vi "CalculateScaleAndPositionToCenterImage.vi"(0 "reference in":refnum<class "LcPictureBox.lvclass">, 2 "ImageFile":path, 3 "Image":refnum<k24>, 5 "Error In":errorcluster) -> (14 "reference out":refnum<class "LcPictureBox.lvclass">, 15 "ScaleFactor":sgl=1.0, 17 "ImagePosition":cluster{"x":sgl, "y":sgl}, 19 "Error Out":errorcluster)   [LabVIEW 2020, in "LcPictureBox.lvclass"]
uses:
  LcPictureBox.lvclass
  System.Drawing
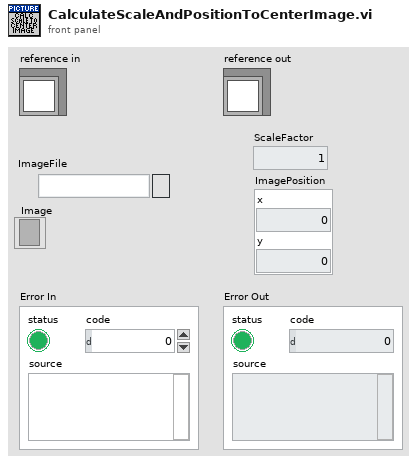
[diagram p1: front panel]
types:
  T1 = typedef "LcPictureBox.lvclass/ObjectAttributes.ctl" = cluster{"PictureBox":refnum<k24>, "ImageSize":cluster{"Width":i32, "Height":i32}, "PenMemory":map{cluster{"Alpha(100%)":dbl, "Color(Black)":u32, "Pen(Width=1, Solid)":T2}, refnum<k24>}, "GraphicsRef":refnum<k24>, "BrushMemory":map{cluster{"Alpha(100%)":dbl, "Color(Black)":u32}, refnum<k24>}, "Images":refnum<k24>[], "ImageIndex":i32, "BgColor(None)":u32, "LoadedImages":map{string, cluster{"ImageOut":refnum<k24>, "ImageSize":cluster{"Width":i32, "Height":i32}}}, "ColorsMemory":map{cluster{"Alpha(100%)":dbl, "Color(Black)":u32}, refnum<k24>}, "CacheSize":i32, "PictureBoxActiveXReference":refnum<vi>, "Scale":sgl, "Offset":cluster{"x":sgl, "y":sgl}, "zoom_center":cluster{"X":i32, "Y":i32}, "ImagesCreated":refnum<k24>[]}
  T2 = typedef "LcPictureBox.lvclass/Pen.ctl" = cluster{"Width":u16, "Style":enum32{"Solid", "Dash", "Dot", "DashDot", "DashDotDot"}}
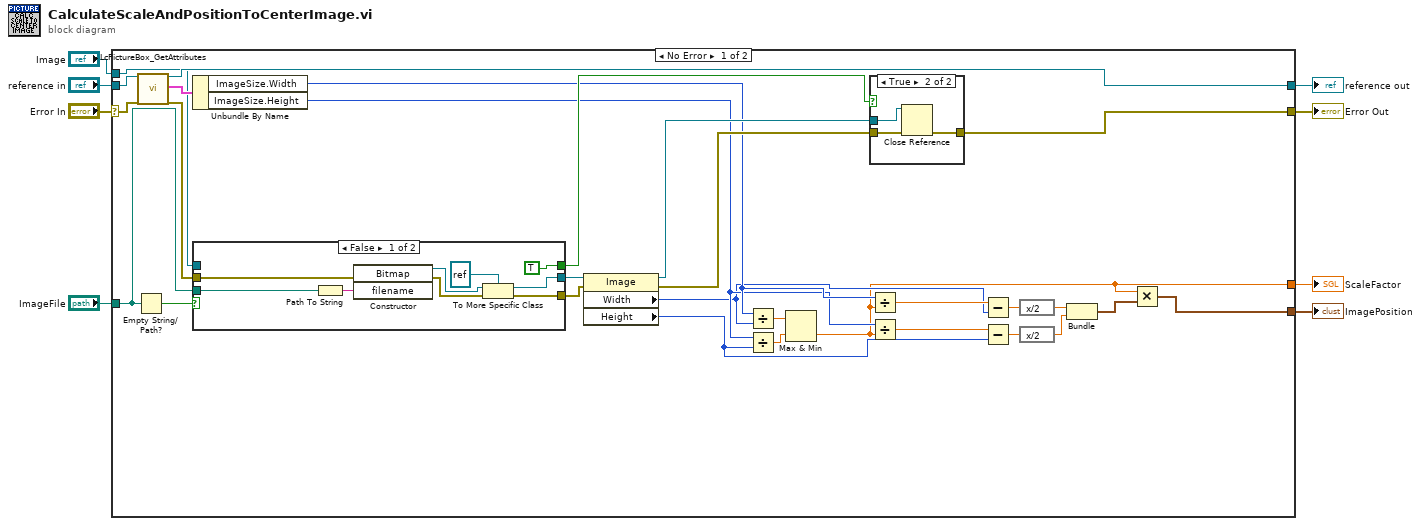
[diagram p0: block diagram]
diagram:
  n1 = case shown="No Error" "Error In" {
    selector: "Error In" -> [w37 w54]
    tunnel: [w20 w54] -> w7
    tunnel: [w34 w53] -> w5
    tunnel: "reference in" -> [w35 w53]
    tunnel: "ImageFile" -> [w32 _]
    tunnel: "Image" -> [w31 _]
    tunnel: [w11 _] -> w2
    tunnel: [w9 _] -> w1
    frame No Error {
      n2 = Empty String/Path?(string/path=w32) -> (empty?=w33:bool)
      n3 = call "LcPictureBox_GetAttributes.vi"("reference in"=w35, "error in (no error)"=w37) -> ("reference out"=w34:refnum<class "LcPictureBox.lvclass">, "Data"=w36:T1, "error out"=w21:errorcluster)  [unwired: 14 in, 1 out]
      n4 = Unbundle By Name(w36) -> ("ImageSize.Width"=w19:i32, "ImageSize.Height"=w18:i32)
      n5 = case shown="False" w33 {
        tunnel: [w47 w51] -> w30
        tunnel: [w46 w52] -> w29
        tunnel: w21 -> [w45 w52]
        tunnel: w32 -> [w43 _]
        tunnel: w31 -> [_ w51]
        tunnel: [TRUE _] -> w28
        frame False {
          n6 = Path To String(path=w43) -> (string=w44:string)
          n7 = constructor class="Bitmap"(error in=w45, "filename"=w44) -> (reference out=w49:refnum<k24>, error out=w48:errorcluster)  [unwired: 2 in, 2 out]
          n8 = To More Specific Class(target class=refnum<k24> refnum, reference=w49, error in=w48) -> (specific class reference=w47:refnum<k24>, error out=w46:errorcluster)
        }
        frame True {
        }
      }
      n9 = property class="Image"(reference=w30, error in=w29) -> (reference out=w27:refnum<k24>, error out=w26:errorcluster, "Width"=w16:i32, "Height"=w13:i32)
      n10 = Divide(x=w19, y=w16) -> (x/y=w25:dbl)
      n11 = Divide(x=w18, y=w13) -> (x/y=w24:dbl)
      n12 = Max & Min(x=w25, y=w24) -> (min(x,y)=w11:dbl)  [unwired: 1 out]
      n13 = case shown="True" w28 {
        tunnel: w27 -> [_ w41]
        tunnel: w26 -> [w38 w40]
        tunnel: [w38 w39] -> w20
        frame False {
        }
        frame True {
          n14 = Close Reference(reference=w41, error in (no error)=w40) -> (error out=w39:errorcluster)
        }
      }
      n15 = Divide(x=w19, y=w11) -> (x/y=w17:dbl)
      n16 = Divide(x=w18, y=w11) -> (x/y=w14:dbl)
      n17 = Subtract(x=w17, y=w16) -> (x-y=w15:dbl)
      n18 = Subtract(x=w14, y=w13) -> (x-y=w12:dbl)
      n19 = expression code="x/2"(w15) -> (w23:dbl)
      n20 = expression code="x/2"(w12) -> (w22:dbl)
      n21 = Bundle(w23, w22) -> (w10:cluster{dbl, dbl})  [unwired: 1 in]
      n22 = Multiply(x=w11, y=w10) -> (x*y=w9:cluster{dbl, dbl})
    }
    frame Error {
    }
  }
  "Error Out" <- w7
  "reference out" <- w5
  "ScaleFactor" <- w2
  "ImagePosition" <- w1
